vi "str-number.vi"(10 "输出数组":T1(array[cluster])) -> (2 "数组":T2(array[cluster]))   [LabVIEW 2016]
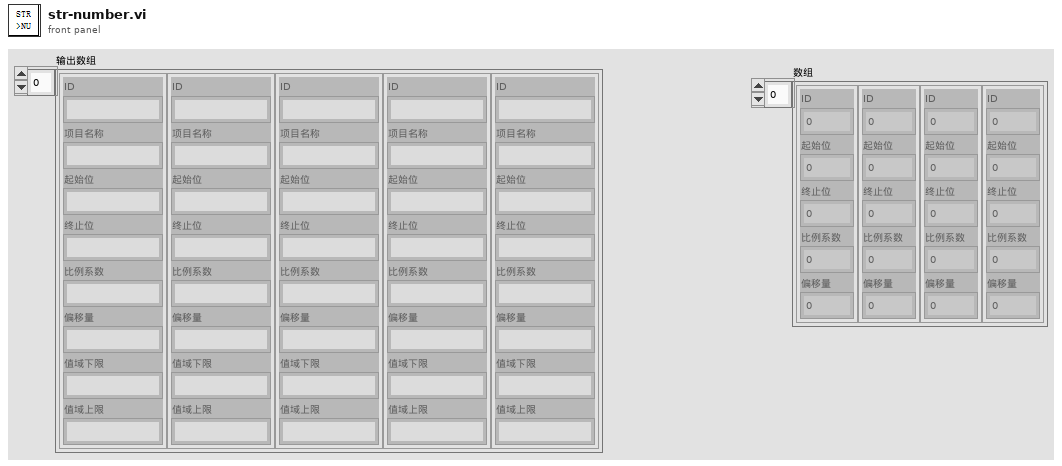
[diagram p1: front panel]
types:
  T1 = cluster{"ID":string, "项目名称":string, "起始位":string, "终止位":string, "比例系数":string, "偏移量":string, "值域下限":string, "值域上限":string}[]
  T2 = cluster{"ID":u32, "起始位":u8, "终止位":u8, "比例系数":dbl, "偏移量":dbl}[]
  T3 = cluster{"ID":u32, "起始位":u8, "终止位":u8, "比例系数":dbl, "偏移量":dbl}
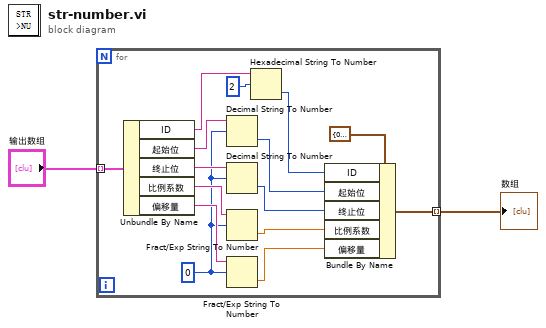
[diagram p0: block diagram]
diagram:
  n1 = for {
    tunnel: [w9] -> w2 mode=indexing
    tunnel: "输出数组" -> [w3] mode=indexing
    w13 = 0
    n2 = Unbundle By Name(w3) -> ("ID"=w12:string, "起始位"=w17:string, "终止位"=w16:string, "比例系数"=w15:string, "偏移量"=w14:string)
    n3 = Decimal String To Number(string=w17, offset=w13) -> (number=w7:i32)  [unwired: 1 in, 1 out]
    n4 = Decimal String To Number(string=w16, offset=w13) -> (number=w6:i32)  [unwired: 1 in, 1 out]
    n5 = Fract/Exp String To Number(string=w15, offset=w13) -> (number=w5:dbl)  [unwired: 2 in, 1 out]
    n6 = Fract/Exp String To Number(string=w14, offset=w13) -> (number=w4:dbl)  [unwired: 2 in, 1 out]
    n7 = Hexadecimal String To Number(string=w12, offset=2 ("偏移量")) -> (number=w8:u32)  [unwired: 1 in, 1 out]
    n8 = Bundle By Name(cluster=T3 {"ID"=0, "起始位"=0, "终止位"=0, "比例系数"=0.0, "偏移量"=0.0} ("簇"), "ID"=w8, "起始位"=w7, "终止位"=w6, "比例系数"=w5, "偏移量"=w4) -> (w9:T3)
  }
  "数组" <- w2
